vi "SV Multitone Gain and Phase (Time) (1 Ch).vi"(0 "response signal [EU]":waveform(dbl), 1 "reference tones":T7(array[cluster]) {"phase (deg)" format="%0.3p"; "amplitude [EU pk]" format="%0.3p"; "frequency [Hz]" format="%0.3p"}, 5 "error in (no error)":errorcluster, 6 "desired units":T8={"gain"=enum."dB", "phase"=enum."deg", "reference level"=enum."EU rms", "response level"=enum."EU rms"}) -> (12 "unit labels":T9, 14 "complex spectrum response":T10={"complex spectrum response"={"f0"=0.0, "df"=1.0, "complex spectrum"=[]}, "spectrum info"={"channel name"="", "description"="", "x-axis units"=0, "spectral info"={"spectrum type"=enum."Power [Magnitude^2]", "linear/dB"=enum."linear", "window"=0, "window size"=0, "FFT size"=0}, "engineering units"=0, "custom label"="", "dB reference [EU]"=0.0, "peak units"=enum."rms", "weighting filter"=0, "spectral density?"=FALSE, "unit label"="", "spectrum skewed?"=FALSE, "complimentary spectrum units"=enum."none"}} {"spectrum info"."x-axis units" items=["Time (s)"=0, "Frequency-CB (Hz)"=1, "Frequency-CPB (Hz)"=1248, "Frequency-Arbitrary (Hz)"=2357, "Quefrency (s)"=2, "Revolutions (rev)"=3, "Order"=4, "Speed (RPM)"=11, "Speed (rad/s)"=21, "Index"=65535]; "spectrum info"."weighting filter" items=["Linear", "A-weighting", "B-weighting", "C-weighting", "ITU-R 468-4", "Dolby", "CCITT", "C-message", "Wb", "Wc", "Wd", "We", "Wf", "Wh", "Wj", "Wk", "Wm", "AES17 20 kHz lowpass", "AES17 40 kHz lowpass", "AES17 20 kHz highpass", "AES17 40 kHz highpass"]; "spectrum info"."dB reference [EU]" format="%.2f"; "spectrum info"."engineering units" items=["custom..."=0, "V"=1, "A"=21, "C"=30, "pC"=31, "s"=32, "-"=29, "Pa"=2, "N"=20, "g"=3, "m/s^2"=4, "m/s"=5, "m"=6, "mm/s"=12, "mm"=13, "micron/s"=14, "micron"=15, "in/s^2"=7, "in/s"=8, "in"=9, "mil/s"=10, "mil"=11, "rad/s^2"=16, "rad/s"=17, "rad"=18, "deg/s^2"=26, "deg/s"=27, "deg"=28, "RPM"=22, "cycle/s^2"=23, "Hz"=24, "cycle"=25, "strain"=19]; "spectrum info"."spectral info"."window" items=["None "=0, "Hanning"=1, "Hamming"=2, "Blackman-Harris"=3, "Exact Blackman"=4, "Blackman"=5, "Flat Top"=6, "4 Term B-Harris "=7, "7 Term B-Harris"=8, "Low Sidelobe"=9, "Force - Exponential"=10, "Gaussian"=62]; "complex spectrum response"."complex spectrum" format="%.2f"; "complex spectrum response"."df" format="%.2f"; "complex spectrum response"."f0" format="%.2f"}, 15 "gain":cluster{"frequency [Hz]":dbl[], "gain":dbl[]} {"gain" format="%_4f"; "frequency [Hz]" format="%.2f"}, 16 "phase":cluster{"frequency [Hz]":dbl[], "phase":dbl[]} {"phase" format="%.2f"; "frequency [Hz]" format="%.2f"}, 17 "gain and phase info":T1={"channel name"="", "description"="", "x-axis units"=0, "spectral info"={"spectrum type"=enum."Power [Magnitude^2]", "linear/dB"=enum."linear", "window"=0, "window size"=0, "FFT size"=0}, "engineering units"=1, "custom label"="", "dB reference [EU]"=0.0, "peak units"=enum."rms", "weighting filter"=0, "spectral density?"=FALSE, "unit label"="", "spectrum skewed?"=FALSE, "complimentary spectrum units"=enum."none"} {"x-axis units" items=["Time (s)"=0, "Frequency-CB (Hz)"=1, "Frequency-CPB (Hz)"=1248, "Frequency-Arbitrary (Hz)"=2357, "Quefrency (s)"=2, "Revolutions (rev)"=3, "Order"=4, "Speed (RPM)"=11, "Speed (rad/s)"=21, "Index"=65535]; "weighting filter" items=["Linear", "A-weighting", "B-weighting", "C-weighting", "ITU-R 468-4", "Dolby", "CCITT", "C-message", "Wb", "Wc", "Wd", "We", "Wf", "Wh", "Wj", "Wk", "Wm", "AES17 20 kHz lowpass", "AES17 40 kHz lowpass", "AES17 20 kHz highpass", "AES17 40 kHz highpass"]; "dB reference [EU]" format="%.2f"; "engineering units" items=["custom..."=0, "V"=1, "A"=21, "C"=30, "pC"=31, "s"=32, "-"=29, "Pa"=2, "N"=20, "g"=3, "m/s^2"=4, "m/s"=5, "m"=6, "mm/s"=12, "mm"=13, "micron/s"=14, "micron"=15, "in/s^2"=7, "in/s"=8, "in"=9, "mil/s"=10, "mil"=11, "rad/s^2"=16, "rad/s"=17, "rad"=18, "deg/s^2"=26, "deg/s"=27, "deg"=28, "RPM"=22, "cycle/s^2"=23, "Hz"=24, "cycle"=25, "strain"=19]; "spectral info"."window" items=["None "=0, "Hanning"=1, "Hamming"=2, "Blackman-Harris"=3, "Exact Blackman"=4, "Blackman"=5, "Flat Top"=6, "4 Term B-Harris "=7, "7 Term B-Harris"=8, "Low Sidelobe"=9, "Force - Exponential"=10, "Gaussian"=62]}, 18 "levels":cluster{"reference":dbl, "response":dbl} {"response" format="%_6f"; "reference" format="%_6f"}, 19 "error out":errorcluster)   [LabVIEW 2017, in "SoundVib_Multitone.lvlib"]
doc: "Use this VI to measure the gain and phase versus frequency. Wire data to <B>scaled signal [EU]</B> to determine the polymorphic instance to use or manually select the instance."
uses:
  <vilib>/addons/Sound and Vibration/svt_Multitone Distortion/SoundVib_Multitone.lvlib
  <vilib>/addons/_NISVFA/_Shared subVIs/Controls/svc_Spectrum Info.ctl
  <vilib>/addons/_NISVFA/_Shared subVIs/Controls/svc_X-Axis Units.ctl
  <vilib>/addons/_NISVFA/_Shared subVIs/Controls/svc_Spectrum Type.ctl
  <vilib>/addons/_NISVFA/_Shared subVIs/Controls/svc_Engineering Units Text Ring.ctl
  <vilib>/addons/_NISVFA/_Shared subVIs/Controls/svc_Weighting Filter Text Ring.ctl
  <vilib>/addons/_NISVFA/_Shared subVIs/Controls/svc_Complimentary Spectrum Units.ctl
  <vilib>/addons/_NISVFA/_Shared subVIs/Controls/svc_Window.ctl
  <vilib>/addons/Sound and Vibration/svt_Distortion/SoundVib_Distortion.lvlib
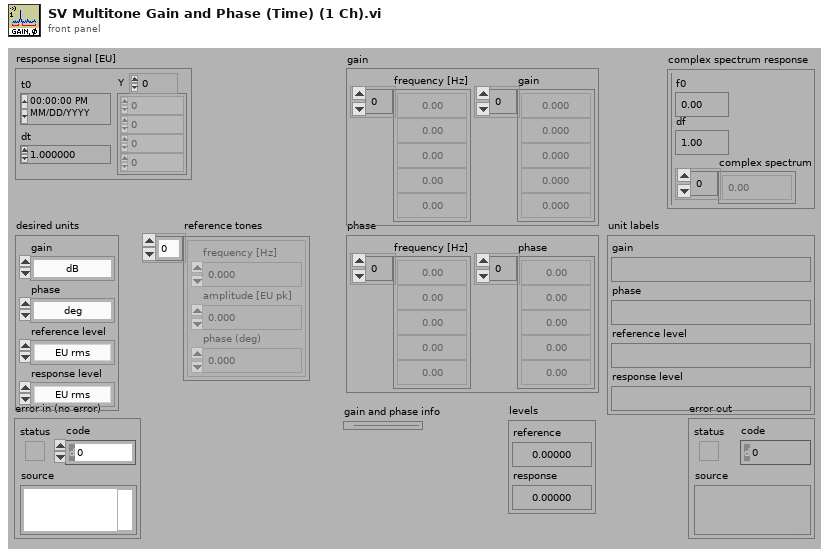
[diagram p1: front panel]
types:
  T1 = typedef "svc_Spectrum Info.ctl" = cluster{"channel name":string, "description":string, "x-axis units":T2, "spectral info":cluster{"spectrum type":T3, "linear/dB":enum16{"linear", "dB"}, "window":u16, "window size":i32, "FFT size":i32}, "engineering units":T4, "custom label":string, "dB reference [EU]":dbl, "peak units":enum16{"rms", "peak", "peak-peak"}, "weighting filter":T5, "spectral density?":bool, "unit label":string, "spectrum skewed?":bool, "complimentary spectrum units":T6}
  T2 = typedef "svc_X-Axis Units.ctl" = u16
  T3 = typedef "svc_Spectrum Type.ctl" = enum16{"FFT Spectrum [complex]", "Amplitude [Magnitude]", "Power [Magnitude^2]", "Cross Spectrum [complex]", "Frequency Response [Complex]"}
  T4 = typedef "svc_Engineering Units Text Ring.ctl" = u16
  T5 = typedef "svc_Weighting Filter Text Ring.ctl" = u16
  T6 = typedef "svc_Complimentary Spectrum Units.ctl" = enum16{"none", "radians", "degrees", "cycles", "imaginary"}
  T7 = cluster{"frequency [Hz]":dbl, "amplitude [EU pk]":dbl, "phase (deg)":dbl}[]
  T8 = cluster{"gain":enum16{"dB", "linear ratio", "%"}, "phase":enum16{"deg", "rad"}, "reference level":enum16{"EU^2 rms", "EU rms", "dB", "dBc", "dBV", "dBu", "dBm"}, "response level":enum16{"EU^2 rms", "EU rms", "dB", "dBc", "dBV", "dBu", "dBm"}}
  T9 = cluster{"gain":string, "phase":string, "reference level":string, "response level":string}
  T10 = cluster{"complex spectrum response":cluster{"f0":dbl, "df":dbl, "complex spectrum":cdb[]}, "spectrum info":T1}
  T11 = typedef "svc_Window.ctl" = u32
  T12 = cluster{"reference level":dbl, "response level":dbl}
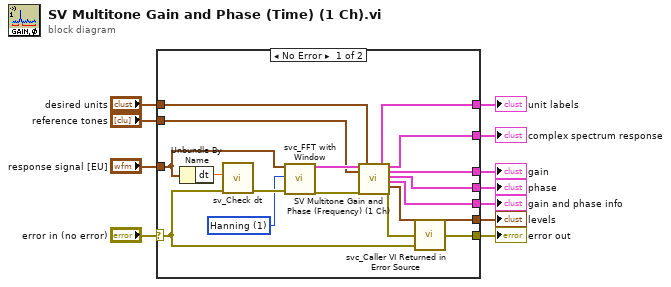
[diagram p0: block diagram]
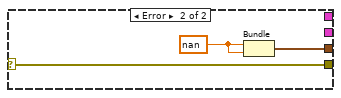
[diagram p2: hidden frame]
diagram:
  n1 = case shown="No Error" "error in (no error)" {
    selector: "error in (no error)" -> [w17 w31]
    tunnel: "response signal [EU]" -> [w19 _]
    tunnel: [w22 w31] -> w10
    tunnel: [w15 _] -> w4
    tunnel: [w16 _] -> w3
    tunnel: [w26 _] -> w8
    tunnel: [w25 _] -> w7
    tunnel: "desired units" -> [w24 _]
    tunnel: [w13 w29] -> w2
    tunnel: "reference tones" -> [w14 _]
    tunnel: [w12 _] -> w1
    frame No Error {
      w20 = T11 1 items=["None ", "Hanning", "Hamming", "Blackman-Harris", "Exact Blackman", "Blackman", "Flat Top", "4 Term B-Harris ", "7 Term B-Harris", "Low Sidelobe", "Force - Exponential", "Gaussian"] ("window")
      n2 = Unbundle By Name(w19) -> ("dt"=w18:dbl)
      n3 = call <vilib>:"sv_Check dt.vi"("error in"=w17, "dt"=w18) -> ("error out"=w21:errorcluster)  [unwired: 8 in, 1 out]
      n4 = call <vilib>:"svc_FFT with Window.vi"("time signal in [EU]"=w19, "window"=w20, "error in (no error)"=w21) -> ("complex spectrum"=w28:T10, "error out"=w27:errorcluster)  [unwired: 15 in]
      n5 = call <vilib>:"SV Multitone Gain and Phase (Frequency) (1 Ch).vi"("complex spectrum response"=w28, "reference tones"=w14, "error in (no error)"=w27, "desired units"=w24) -> ("unit labels"=w26:T9, "complex spectrum response"=w25:T10, "gain"=w15:cluster{"frequency [Hz]":dbl[], "gain":dbl[]}, "phase"=w16:cluster{"frequency [Hz]":dbl[], "phase":dbl[]}, "gain and phase info"=w12:T1, "levels"=w13:T12, "error out"=w23:errorcluster)  [unwired: 9 in]
      n6 = call <vilib>:"svc_Caller VI Returned in Error Source.vi"("warning input to caller"=w17, "error in (no error)"=w23) -> ("error out"=w22:errorcluster)  [unwired: 3 in]
    }
    frame Error {
      w30 = nan ("SINAD")
      n7 = Bundle("SINAD"=w30, "SINAD"=w30) -> (w29:cluster{"SINAD":dbl, "SINAD":dbl})  [unwired: 1 in]
    }
  }
  "error out" <- w10
  "phase" <- w3
  "levels" <- w2
  "complex spectrum response" <- w7
  "unit labels" <- w8
  "gain" <- w4
  "gain and phase info" <- w1
